vi "Initialize New.vi"(8 "error in (no error)":errorcluster, 10 "count":i32, 11 "Core Transfers Configuration in":refnum<class "Core Transfers Configuration.lvclass">) -> (0 "error out":errorcluster, 3 "Core Transfers Configuration out":refnum<class "Core Transfers Configuration.lvclass">)   [LabVIEW 2017, in "DSF Core.lvlib" / "Core Transfers Configuration.lvclass"]
uses:
  Core Transfers Configuration.lvclass
  Configuration.ctl
  Core Transfers Configuration.lvclass/Core Transfers Configuration.ctl
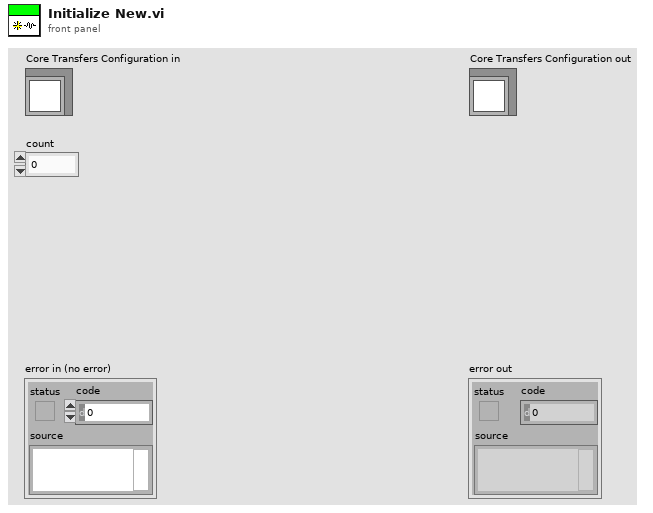
[diagram p1: front panel]
types:
  T1 = typedef "DSF Core.lvlib/Core Transfers Configuration.lvclass/Configuration.ctl" = cluster{"name":string}
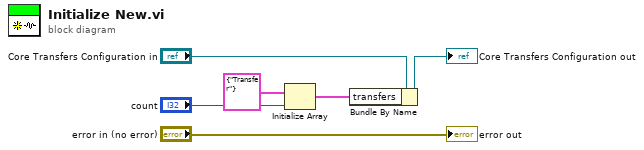
[diagram p0: block diagram]
diagram:
  n1 = Initialize Array(T1 {"name"="Transfer"} ("transfers"), "count") -> (w2:T1[])
  n2 = Bundle By Name(cluster="Core Transfers Configuration in", "transfers"=w2) -> (→"Core Transfers Configuration out":refnum<class "Core Transfers Configuration.lvclass">)
  "error out" <- "error in (no error)"
